vi "User Console View.vi"(8 "error in (no error)":errorcluster, 11 "View Model":T1) -> (0 "error out":errorcluster)   [LabVIEW 2017]
doc: "The interface where a user calls the Elevator, makes a floor selection, and reports an Emergency.\n[Covers: UI2]"
uses:
  View Model/Controls/View Model.ctl
  View Model/Controls/Shared Model.ctl
  Error/Controls/Error Model.ctl
  Error/Controls/Error Event.ctl
  Error/Controls/Error Type.ctl
  Configuration/Controls/Config DB Model.ctl
  Configuration/Controls/Config DB Command.ctl
  Configuration/Controls/Config DB Record.ctl
  Controller/Controls/Controller Model.ctl
  Controller/Controls/Elevator Location.ctl
  Controller/Controls/Elevator Direction Event.ctl
  Controller/Controls/Elevator Direction.ctl
  Controller/Controls/Elevator CMD Event.ctl
  Controller/Controls/Elevator Commands.ctl
  Controller/Controls/Elevator Overhead.ctl
  Controller/Controls/Elevator State.ctl
  Controls/User Console - GUI refs.ctl
panel:
  in  "Emergency":bool
  in  "Open Door":bool
  in  "Close Door":bool
  in  "1st Floor":bool
  in  "2nd Floor":bool
  in  "3rd Floor":bool
  in  "4th Floor":bool
  in  "Up 1":bool
  in  "Up 2":bool
  in  "Up 3":bool
  in  "Down 2":bool
  in  "Down 3":bool
  in  "Down 4":bool
  # "Elevator Call"
  # "Floor Selection"
  # "Fourth Floor"
  # "Third Floor"
  # "Second Floor"
  # "First Floor"
  # "[Covers: UI2A]"
  # "[Covers: UI2B]"
  # "[Covers: UI2B2]"
  # "[Covers: UI2A1]"
  # "[Covers: UI2A2]"
  # "Door Buttons"
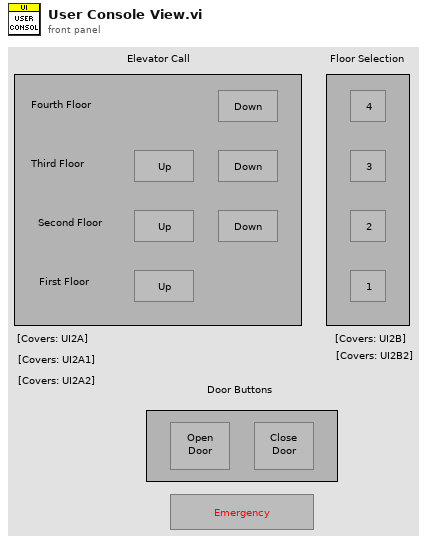
[diagram p1: front panel]
types:
  T1 = typedef "View Model.ctl" = cluster{"Shared Model":T2, "Error Model":T3, "Config Model":T4, "Controller Model":T5}
  T2 = typedef "Shared Model.ctl" = cluster{"Stop":refnum<user-event>, "Stop DVR":refnum<data-value>}
  T3 = typedef "Error Model.ctl" = cluster{"Error":refnum<user-event>}
  T4 = typedef "Config DB Model.ctl" = cluster{"DB Command":refnum<user-event>, "DB Record DVR":refnum<data-value>}
  T5 = typedef "Controller Model.ctl" = cluster{"Go to Floor":refnum<user-event>, "Emergency":refnum<user-event>, "Open/Close Door":refnum<user-event>, "Move To":refnum<user-event>, "Position Change":refnum<user-event>, "Elevator CMD Event":refnum<user-event>, "Overhead DVR":refnum<data-value>, "Motion Event":refnum<user-event>}
  T6 = typedef "User Console - GUI refs.ctl" = cluster{"1 st Floor":refnum<vi>, "2 nd Floor":refnum<vi>, "3 rd Floor":refnum<vi>, "4 th Floor":refnum<vi>, "Up 1":refnum<vi>, "Up 2":refnum<vi>, "Up 3":refnum<vi>, "Down 2":refnum<vi>, "Down 3":refnum<vi>, "Down 4":refnum<vi>, "Open Door":refnum<vi>, "Close Door":refnum<vi>, "Emergency":refnum<vi>}
  T7 = typedef "Elevator Location.ctl" = enum16{"1st Floor", "2nd Floor", "3rd Floor", "4th Floor"}
  T8 = typedef "Elevator State.ctl" = enum16{"No Request", "Initial", "Wait for 1st Request", "Start and Move", "Anakysis", "Continue Travel", "Stop at Floor", "Open/Close Door", "Emergency", "Terminate"}
  T9 = typedef "Elevator Commands.ctl" = enum16{"Go Up", "Go Down", "Go to Floor", "Emergency", "Open Doors", "Close Doors"}
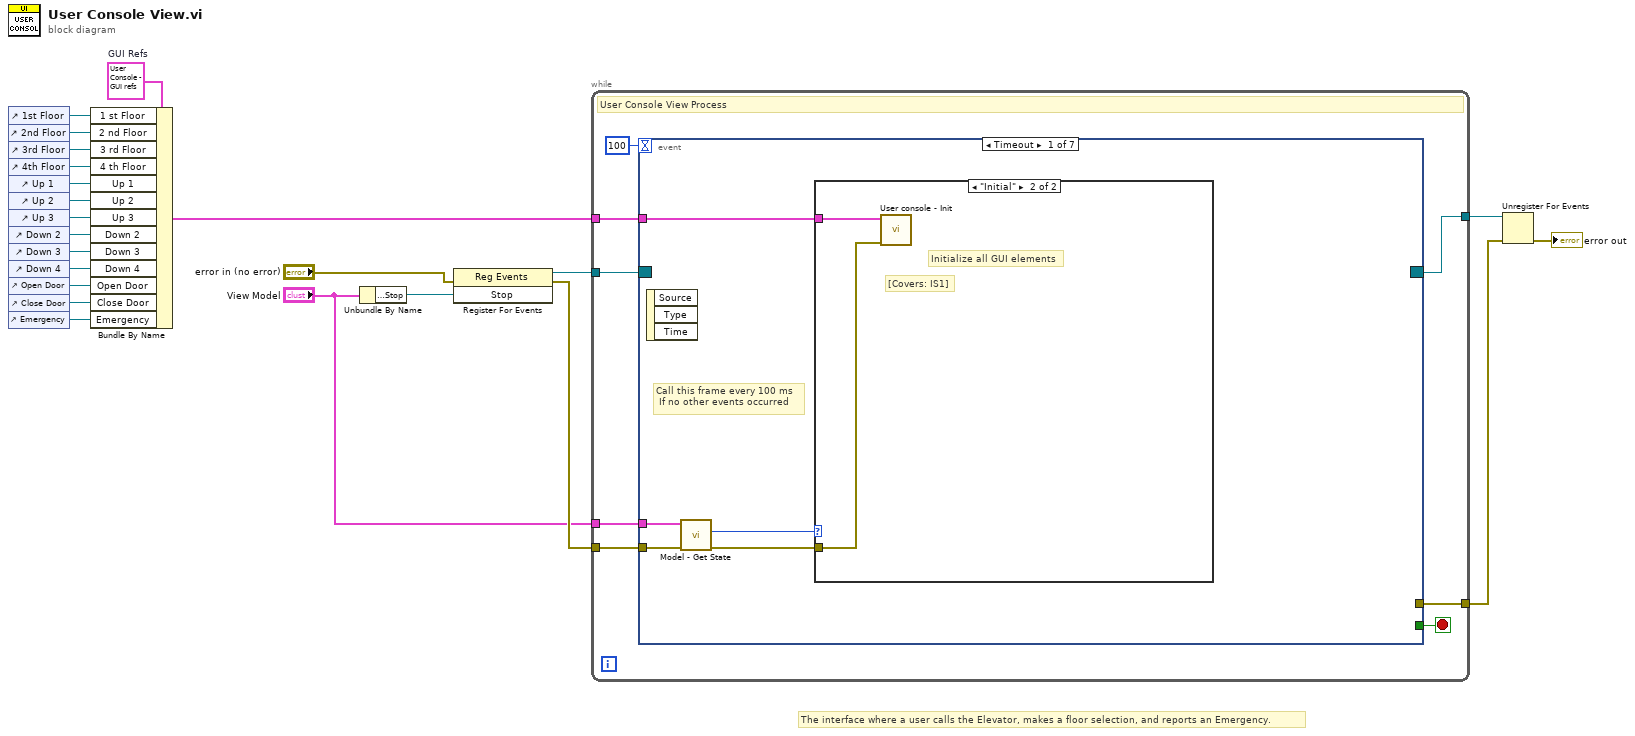
[diagram p0: block diagram]
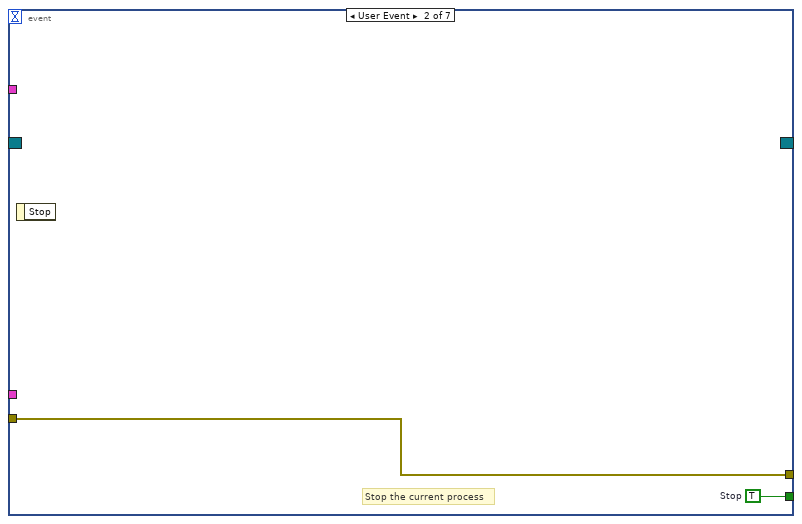
[diagram p3: hidden frame]
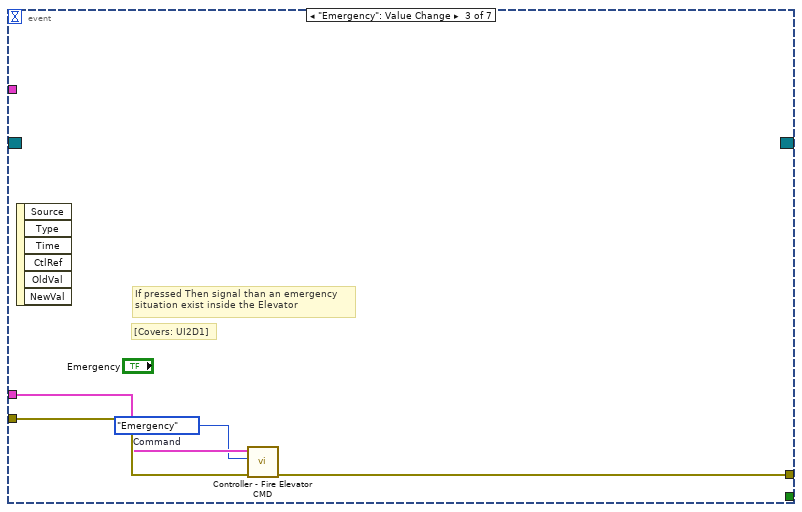
[diagram p4: hidden frame]
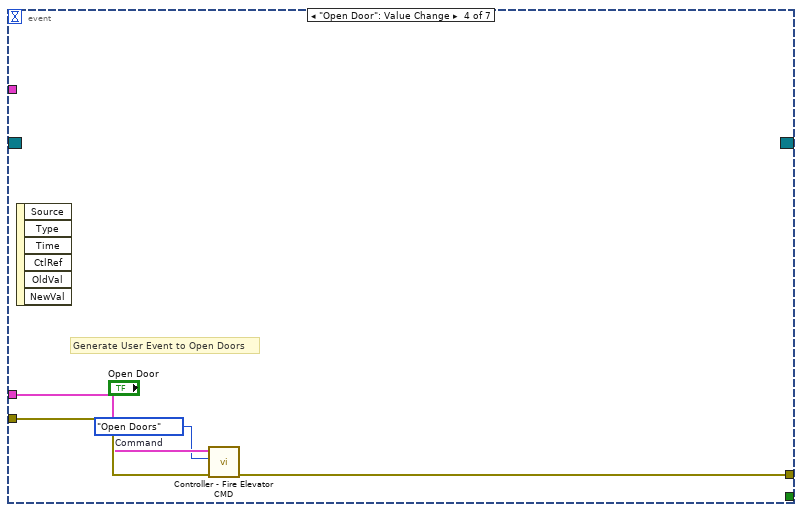
[diagram p5: hidden frame]
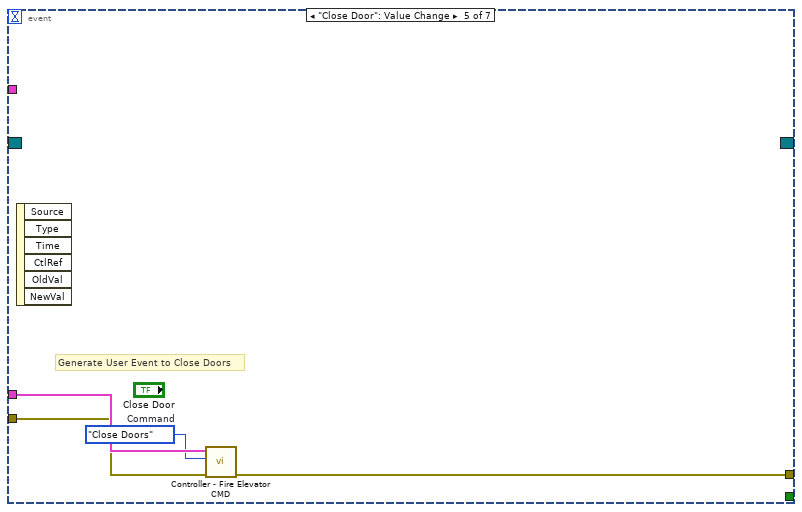
[diagram p6: hidden frame]
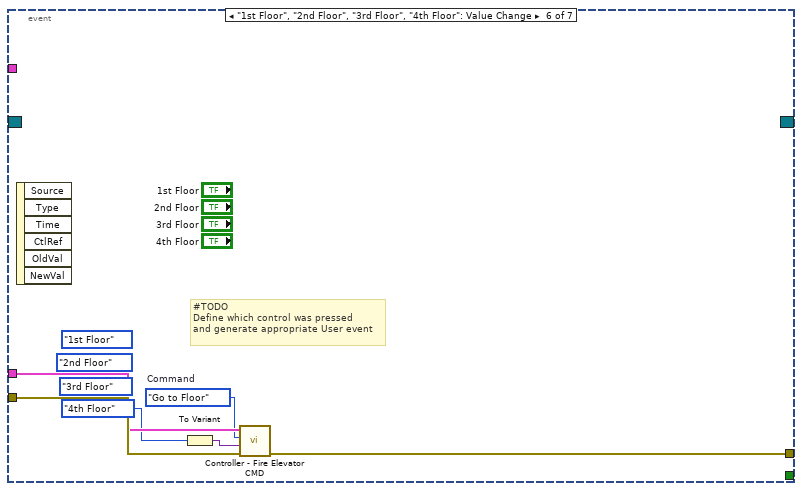
[diagram p7: hidden frame]
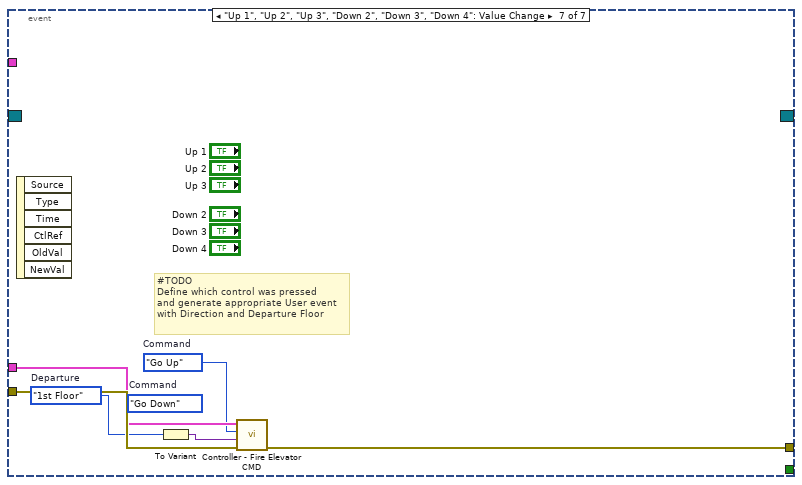
[diagram p8: hidden frame]
diagram:
  w15 = T6 {"1 st Floor"=refnum, "2 nd Floor"=refnum, "3 rd Floor"=refnum, "4 th Floor"=refnum, "Up 1"=refnum, "Up 2"=refnum, "Up 3"=refnum, "Down 2"=refnum, "Down 3"=refnum, "Down 4"=refnum, "Open Door"=refnum, "Close Door"=refnum, "Emergency"=refnum}  # GUI Refs
  # "The interface where a user calls the Elevator, makes a floor selection, and reports an Emergency."
  n1 = control-ref of="1st Floor"() -> (w14:refnum<vi>)
  n2 = control-ref of="2nd Floor"() -> (w2:refnum<vi>)
  n3 = control-ref of="3rd Floor"() -> (w3:refnum<vi>)
  n4 = control-ref of="4th Floor"() -> (w4:refnum<vi>)
  n5 = control-ref of="Up 1"() -> (w5:refnum<vi>)
  n6 = control-ref of="Up 2"() -> (w6:refnum<vi>)
  n7 = control-ref of="Up 3"() -> (w7:refnum<vi>)
  n8 = control-ref of="Down 2"() -> (w8:refnum<vi>)
  n9 = control-ref of="Down 3"() -> (w9:refnum<vi>)
  n10 = control-ref of="Down 4"() -> (w10:refnum<vi>)
  n11 = control-ref of="Open Door"() -> (w11:refnum<vi>)
  n12 = control-ref of="Close Door"() -> (w12:refnum<vi>)
  n13 = control-ref of="Emergency"() -> (w13:refnum<vi>)
  n14 = Bundle By Name(cluster=w15, "1 st Floor"=w14, "2 nd Floor"=w2, "3 rd Floor"=w3, "4 th Floor"=w4, "Up 1"=w5, "Up 2"=w6, "Up 3"=w7, "Down 2"=w8, "Down 3"=w9, "Down 4"=w10, "Open Door"=w11, "Close Door"=w12, "Emergency"=w13) -> (w1:T6)
  n15 = Unbundle By Name("View Model") -> ("Shared Model.Stop"=w23:refnum<user-event>)
  n16 = register-events(error in="error in (no error)", w23) -> (reference out=w22:refnum<event-registration>, error out=w19:errorcluster)  [unwired: 1 in]
  n17 = while {
    tunnel: w22 -> [w31]
    tunnel: [w30] -> w21
    tunnel: w19 -> [w29]
    tunnel: "View Model" -> [w28]
    tunnel: [w27] -> w17
    tunnel: w1 -> [w24]
    stop <- w26 stop-if-true
    # "User Console View Process"
    n18 = event shown="[0] Timeout" {
      selector: w31 -> [_ _ _ _ _ _ _]
      dyn-events: [_ _ _ _ _ _ _] -> w30
      timeout: 100 -> [_ _ _ _ _ _ _]
      tunnel: w29 -> [w36 w40 w44 w48 w51 w58 w64]
      tunnel: w28 -> [w35 _ w43 w47 w52 w57 w63]
      tunnel: [_ w40 w42 w46 w50 w56 w62] -> w27
      tunnel: [_ w39 _ _ _ _ _] -> w26
      tunnel: w24 -> [w33 _ _ _ _ _ _]
      event Timeout {
        # "Call this frame every 100 ms\n If no other events occurred"
        n19 = event-data() -> ()  [unwired: 1 in, 3 out]
        n20 = call "Model - Get State.vi"("error in (no error)"=w36, "View Model"=w35) -> ("error out"=w32:errorcluster, "Current State"=w34:T8)  [unwired: 6 in, 2 out]
        n21 = case shown="\"Initial\"" w34 {
          tunnel: w33 -> [_ w38]
          tunnel: w32 -> [_ w37]
          frame Default {
          }
          frame "Initial" {
            # "Initialize all GUI elements"
            # "[Covers: IS1]"
            n22 = call "User console - Init.vi"("error in (no error)"=w37, "GUI Refs"=w38) -> ()  [unwired: 9 in, 1 out]
          }
        }
      }
      event User Event {
        w39 = TRUE  # Stop
        # "Stop the current process"
        n23 = event-data() -> ()  [unwired: 1 in, 1 out]
      }
      event "Emergency": Value Change {
        w41 = Elevator_Commands."Emergency"  # Command
        # "[Covers: UI2D1]"
        # "If pressed Then signal than an emergency\nsituation exist inside the Elevator"
        n24 = event-data() -> ()  [unwired: 1 in, 6 out]
        n25 = call "Controller - Fire Elevator CMD.vi"("error in (no error)"=w44, "Command"=w41, "View Model"=w43) -> ("error out"=w42:errorcluster)  [unwired: 7 in, 1 out]
      }
      event "Open Door": Value Change {
        w45 = Elevator_Commands."Open Doors"  # Command
        # "Generate User Event to Open Doors"
        n26 = event-data() -> ()  [unwired: 1 in, 6 out]
        n27 = call "Controller - Fire Elevator CMD.vi"("error in (no error)"=w48, "Command"=w45, "View Model"=w47) -> ("error out"=w46:errorcluster)  [unwired: 7 in, 1 out]
      }
      event "Close Door": Value Change {
        w49 = Elevator_Commands."Close Doors"  # Command
        # "Generate User Event to Close Doors"
        n28 = event-data() -> ()  [unwired: 1 in, 6 out]
        n29 = call "Controller - Fire Elevator CMD.vi"("error in (no error)"=w51, "Command"=w49, "View Model"=w52) -> ("error out"=w50:errorcluster)  [unwired: 7 in, 1 out]
      }
      event "1st Floor", "2nd Floor", "3rd Floor", "4th Floor": Value Change {
        w55 = Elevator_Commands."Go to Floor"  # Command
        (unwired) Elevator_Location."3rd Floor" ("Destination")
        (unwired) Elevator_Location."2nd Floor" ("Destination")
        (unwired) Elevator_Location."1st Floor" ("Destination")
        # "#TODO\nDefine which control was pressed\nand generate appropriate User event"
        n30 = event-data() -> ()  [unwired: 1 in, 6 out]
        n31 = To Variant(anything=Elevator_Location."4th Floor" ("Destination")) -> (Variant=w53:variant)
        n32 = call "Controller - Fire Elevator CMD.vi"("error in (no error)"=w58, "Data"=w53, "Command"=w55, "View Model"=w57) -> ("error out"=w56:errorcluster)  [unwired: 6 in, 1 out]
      }
      event "Up 1", "Up 2", "Up 3", "Down 2", "Down 3", "Down 4": Value Change {
        (unwired) Elevator_Commands."Go Down"  # Command
        w60 = Elevator_Location."1st Floor"  # Departure
        w61 = Elevator_Commands."Go Up"  # Command
        # "#TODO\nDefine which control was pressed\nand generate appropriate User event\nwith Direction and Departure Floor"
        n33 = event-data() -> ()  [unwired: 1 in, 6 out]
        n34 = To Variant(anything=w60) -> (Variant=w59:variant)
        n35 = call "Controller - Fire Elevator CMD.vi"("error in (no error)"=w64, "Data"=w59, "Command"=w61, "View Model"=w63) -> ("error out"=w62:errorcluster)  [unwired: 6 in, 1 out]
      }
    }
  }
  n36 = Unregister For Events(event registration refnum=w21, error in=w17) -> (error out=→"error out":errorcluster)
